vi "Dual Operators.vi"   [LabVIEW 2019]
uses:
  Robot Global Data.vi
types:
  T1 = typedef "WPI_JoystickDevRef.ctl" = cluster{"Device":T2}
  T2 = typedef "WPI_JoystickDeviceEnum.ctl" = enum16{"USB 0", "USB 1", "USB 2", "USB 3", "USB 4", "USB 5"}
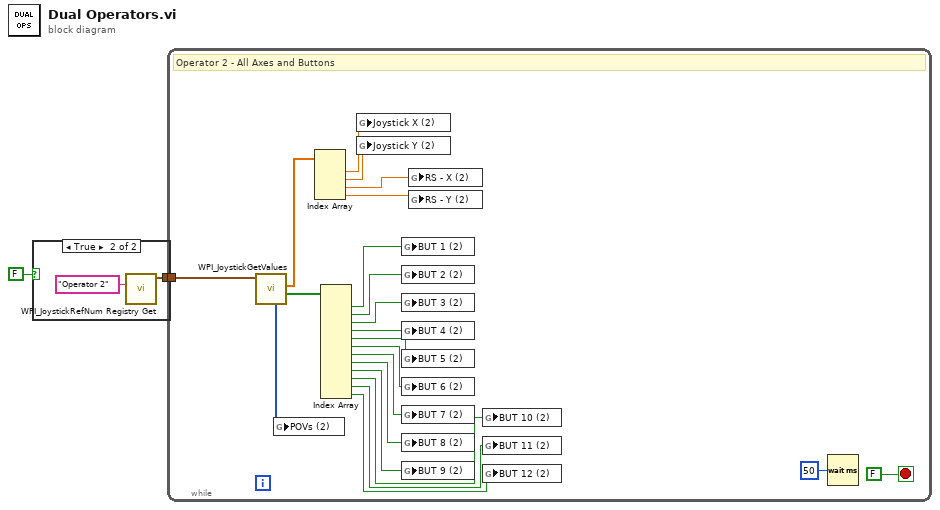
[diagram p0: block diagram]
diagram:
  n1 = case shown="True" FALSE {
    tunnel: [_ w3] -> w1
    frame False {
    }
    frame True {
      n2 = call <vilib>:"WPI_JoystickRefNum Registry Get.vi"("refnum name"="Operator 2") -> ("JoystickDevRef"=w3:T1)  [unwired: 1 in, 9 out]
    }
  }
  n3 = while {
    tunnel: w1 -> [w10]
    stop <- FALSE stop-if-true
    # "Operator 2 - All Axes and Buttons"
    n4 = call <vilib>:"WPI_JoystickGetValues.vi"("JoystickDevRef"=w10) -> ("Buttons"=w12:bool[], "Axes"=w9:dbl[], "POVs"=w11:i16[])  [unwired: 6 in, 2 out]
    n5 = global write "Robot Global Data.vi" "POVs (2)"(w11) -> ()
    n6 = Index Array(array=w9) -> (element #1=w8:dbl, element #2=w7:dbl, element #3=w6:dbl, element #4=w5:dbl)  [unwired: 4 in]
    n7 = Index Array(array=w12) -> (element #1=w13:bool, element #2=w14:bool, element #3=w15:bool, element #4=w16:bool, element #5=w17:bool, element #6=w18:bool, element #7=w19:bool, element #8=w20:bool, element #9=w21:bool, element #10=w22:bool, element #11=w23:bool, element #12=w24:bool)  [unwired: 12 in]
    n8 = global write "Robot Global Data.vi" "Joystick X (2)"(w8) -> ()
    n9 = global write "Robot Global Data.vi" "Joystick Y (2)"(w7) -> ()
    n10 = global write "Robot Global Data.vi" "BUT 1 (2)"(w13) -> ()
    n11 = global write "Robot Global Data.vi" "BUT 2 (2)"(w14) -> ()
    n12 = global write "Robot Global Data.vi" "BUT 3 (2)"(w15) -> ()
    n13 = global write "Robot Global Data.vi" "BUT 4 (2)"(w16) -> ()
    n14 = global write "Robot Global Data.vi" "BUT 5 (2)"(w17) -> ()
    n15 = global write "Robot Global Data.vi" "BUT 6 (2)"(w18) -> ()
    n16 = global write "Robot Global Data.vi" "BUT 7 (2)"(w19) -> ()
    n17 = global write "Robot Global Data.vi" "BUT 8 (2)"(w20) -> ()
    n18 = global write "Robot Global Data.vi" "BUT 9 (2)"(w21) -> ()
    n19 = global write "Robot Global Data.vi" "RS - X (2)"(w6) -> ()
    n20 = global write "Robot Global Data.vi" "RS - Y (2)"(w5) -> ()
    n21 = global write "Robot Global Data.vi" "BUT 10 (2)"(w22) -> ()
    n22 = global write "Robot Global Data.vi" "BUT 11 (2)"(w23) -> ()
    n23 = global write "Robot Global Data.vi" "BUT 12 (2)"(w24) -> ()
    n24 = Wait (ms)(milliseconds to wait=u32 50) -> ()  [unwired: 1 out]
  }
